vi "SPC_get_fifo_init_vars.vi"(8 "Error In":errorcluster, 10 "Module No.":i16, 11 "DLL Path":path) -> (0 "Error Out":errorcluster, 1 "spc_header":u32 max=127 step=1 format="%x", 2 "Module No.":i16, 3 "DLL Path":path, 4 "mt_clock ( 0.1 ns units)":i32, 5 "Fifo Type":T1=7 items=["48 bits SPC-6x0"=2, "32 bits SPC-6x0"=3, "32 bits SPC-130"=4, "32 bits SPC-830"=5, "32 bits SPC-140"=6, "32 bits SPC-150"=7, "32 bits DPC-230"=8, "32 bits FIFO_IMAGE"=9, "FIFO_D590"=10, "FIFO_TDC"=11, "FIFO_TDC_ABS"=12], 7 "stream_type":i16=1 max=1536 step=1 format="%x")   [LabVIEW 2019]
doc: "This procedure sets variables to be used as input parameters for SPC_init_buf_stream function.\nIt can also prepare .spc file header ( 1st word of .spc file), if saving .spc files is required. \nThe procedure is intended to be used directly before starting FIFO measurement to initialize a'buffered' stream.\nIf photons are added to the stream not from running FIFO measurement, but e.g. .spc files, then input parameters for SPC_init_buf_stream must be taken from .spc file header.\n\ninfo@becker-hickl.com"
uses:
  SPC_Controls/Fifo_Type.ctl
panel:
  out "fifo_type":i16
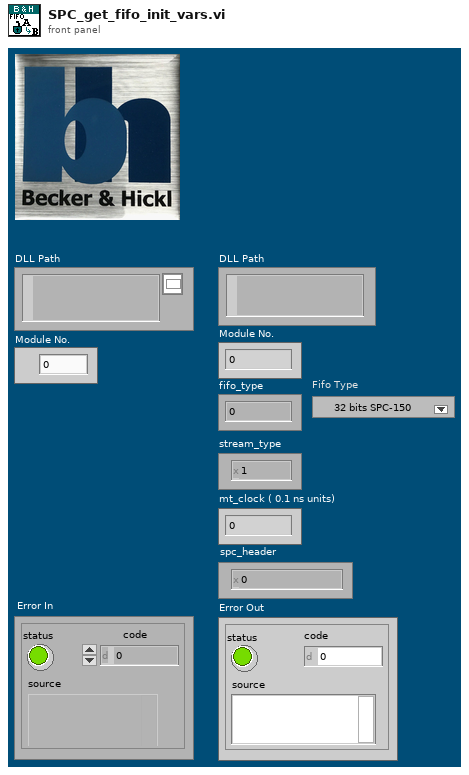
[diagram p1: front panel]
types:
  T1 = typedef "Fifo_Type.ctl" = i16
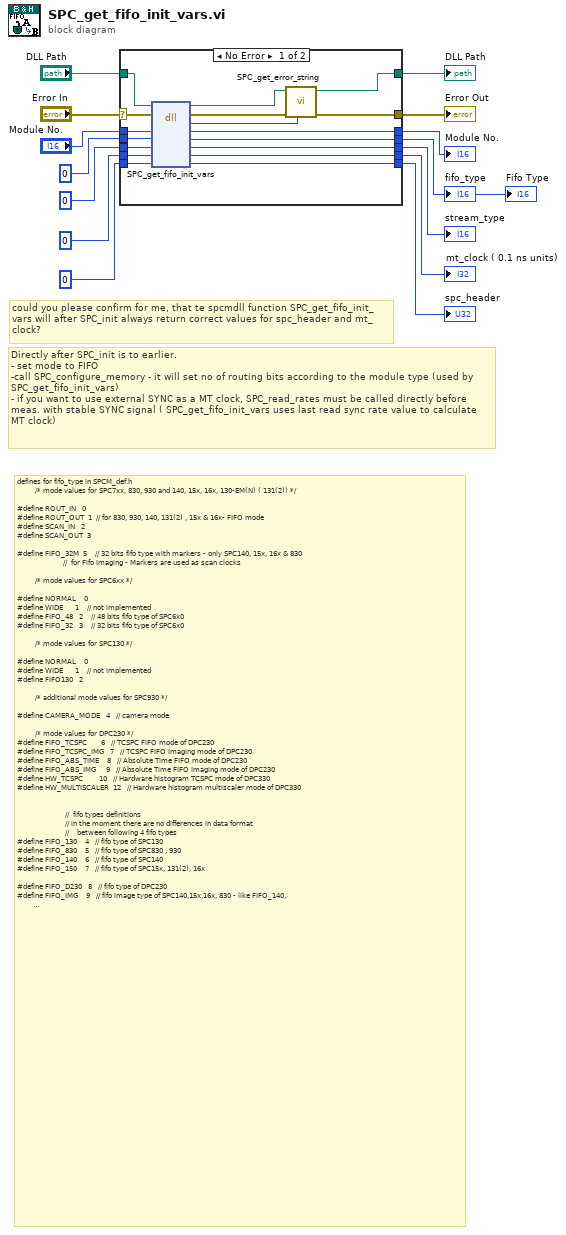
[diagram p0: block diagram]
diagram:
  # "defines for fifo_type in SPCM_def.h\n         /* mode values for SPC7xx, 830, 930 and 140, 15x, 16x, 130-EM(N) ( 131(2)) */\n         \n#define ROUT_IN   0           \n#define ROUT_OUT  1  // for 830, 930, 140, 131(2) , 15x & 16x- FIFO mode         \n#define SCAN_IN   2           \n#define SCAN_OUT  3           \n         \n#define FIFO_32M  5    // 32 bits fifo type with markers - only SPC140, 15x, 16x & 830\n                       //  for Fifo Imaging - Markers are used as scan clocks\n                       \n         /* mode values for SPC6xx */\n         \n#define NORMAL    0           \n#define WIDE      1    // not implemented\n#define FIFO_48   2    // 48 bits fifo type of SPC6x0       \n#define FIFO_32   3    // 32 bits fifo type of SPC6x0        \n\n         /* mode values for SPC130 */\n         \n#define NORMAL    0           \n#define WIDE      1    // not implemented\n#define FIFO130   2           \n\n         /* additional mode values for SPC930 */\n         \n#define CAMERA_MODE   4   // camera mode\n\n         /* mode values for DPC230 */\n#define FIFO_TCSPC       6   // TCSPC FIFO mode of DPC230\n#define FIFO_TCSPC_IMG   7   // TCSPC FIFO Imaging mode of DPC230\n#define FIFO_ABS_TIME    8   // Absolute Time FIFO mode of DPC230\n#define FIFO_ABS_IMG     9   // Absolute Time FIFO Imaging mode of DPC230\n#define HW_TCSPC        10   // Hardware histogram TCSPC mode of DPC330\n#define HW_MULTISCALER  12   // Hardware histogram multiscaler mode of DPC330\n\n\n                        //  fifo types definitions\n                        // in the moment there are no differences in data format\n                        //    between following 4 fifo types\n#define FIFO_130    4   // fifo type of SPC130\n#define FIFO_830    5   // fifo type of SPC830 , 930\n#define FIFO_140    6   // fifo type of SPC140\n#define FIFO_150    7   // fifo type of SPC15x, 131(2), 16x\n\n#define FIFO_D230   8   // fifo type of DPC230\n#define FIFO_IMG    9   // fifo image type of SPC140,15x,16x, 830 - like FIFO_140, \n                        //      but with marker photons\n#define FIFO_D590   10  // fifo type of DPC590"
  # "Directly after SPC_init is to earlier.\n- set mode to FIFO\n-call SPC_configure_memory - it will set no of routing bits according to the module type (used by SPC_get_fifo_init_vars)\n- if you want to use external SYNC as a MT clock, SPC_read_rates must be called directly before meas. with stable SYNC signal ( SPC_get_fifo_init_vars uses last read sync rate value to calculate MT clock)"
  # "could you please confirm for me, that te spcmdll function SPC_get_fifo_init_vars will after SPC_init always return correct values for spc_header and mt_clock?"
  n1 = case shown="No Error" "Error In" {
    selector: "Error In" -> [w29 w38]
    tunnel: "DLL Path" -> [w31 w37]
    tunnel: [w16 w37] -> w13
    tunnel: [w28 w38] -> w11
    tunnel: "Module No." -> [w26 w36]
    tunnel: [w25 w36] -> w9
    tunnel: [w24 w32] -> w1
    tunnel: [w23 w35] -> w8
    tunnel: i16 0 ("Stream type") -> [w22 w35]
    tunnel: [w21 w34] -> w6
    tunnel: 0 ("MT clock ( 0.1 ns units)") -> [w20 w34]
    tunnel: [w19 w33] -> w4
    tunnel: u32 0 ("SPC Header") -> [w18 w33]
    tunnel: i16 0 ("fifo_type") -> [w15 w32]
    frame No Error {
      n2 = dll-call lib="D:/spcm/lib/lab_view/lv10.0/spcm32.dll" fn="SPC_get_fifo_init_vars"(path in=w31, error in=w29, "mod_no"=w26, "fifo_type"=w15, "stream_type"=w22, "mt_clock"=w20, "spc_header"=w18) -> (path out=w17:path, error out=w30:errorcluster, "return type"=w27:i16, "mod_no"=w25:i16, "fifo_type"=w24:i16, "stream_type"=w23:i16, "mt_clock"=w21:i32, "spc_header"=w19:u32)  [unwired: 1 in]
      n3 = call "SPC_get_error_string.vi"("ErrorID"=w27, "Error In"=w30, "DLL Path"=w17) -> ("Error Out"=w28:errorcluster, "DLL Path"=w16:path)  [unwired: 6 in, 1 out]
    }
    frame Error {
    }
  }
  "DLL Path" <- w13
  "Error Out" <- w11
  "Module No." <- w9
  "stream_type" <- w8
  "mt_clock ( 0.1 ns units)" <- w6
  "spc_header" <- w4
  "fifo_type" <- w1
  "Fifo Type" <- w1
